vi "GET PARABOLIC FIT POINTS.vi"(7 "Data entry":u16(ring) items=["Points N°", "Frequency (kHz)", "% of span"], 8 "Sweep size":u32=1000, 9 "F stop":u32=2000500, 10 "F start":u32=200000, 11 "Parabolic fit span":u32) -> (3 "Points":i32)   [LabVIEW 2021]
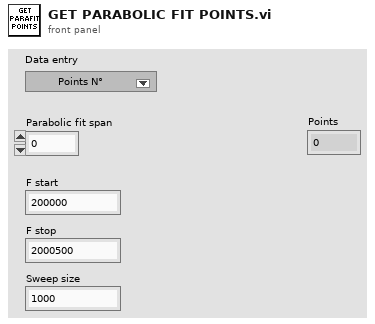
[diagram p1: front panel]
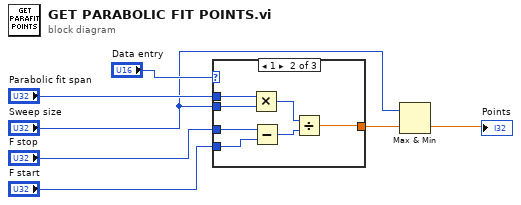
[diagram p0: block diagram]
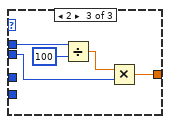
[diagram p3: hidden frame]
diagram:
  n1 = case shown="1" "Data entry" {
    tunnel: "Parabolic fit span" -> [w8 w13 w20]
    tunnel: [w8 w9 w17] -> w1
    tunnel: "Sweep size" -> [_ w12 w16]
    tunnel: "F stop" -> [_ w15 _]
    tunnel: "F start" -> [_ w14 _]
    frame 0, Default {
    }
    frame 1 {
      n2 = Multiply(x=w13, y=w12) -> (x*y=w11:u32)
      n3 = Subtract(x=w15, y=w14) -> (x-y=w10:u32)
      n4 = Divide(x=w11, y=w10) -> (x/y=w9:dbl)
    }
    frame 2 {
      n5 = Divide(x=w20, y=u32 100) -> (x/y=w18:dbl)
      n6 = Multiply(x=w18, y=w16) -> (x*y=w17:dbl)
    }
  }
  n7 = Max & Min(x="Sweep size", y=w1) -> (min(x,y)=→"Points":dbl)  [unwired: 1 out]
